vi "Spectrometer_hittite.vi"(6 "ESR_stack_ref":refnum<vi>, 8 "current_run_ref":refnum<vi>, 9 "generator_enable":bool, 10 "sweep_parameters":T2={"Repetitions"=1, "Power dBm"=5.999999061226845, "Freq Start [Hz]"=2800000000.0, "Freq Stop [Hz]"=3000000000.0, "Step size [Hz]"=2500000.0, "Dwell Time [s]"=0.09999999974525053} {"Dwell Time [s]" format="%.3f"; "Step size [Hz]" format="%.2p"; "Freq Stop [Hz]" format="%.2p"; "Freq Start [Hz]" format="%.2p"; "Power dBm" format="%.2f"; "Repetitions" min=1 max=1000 step=1}, 11 "position_xyz":T1 {"Position Z" min=0.0 max=10.0 step=0.001 format="%.3f"; "Position Y" min=-10.0 max=10.0 step=0.1 format="%.3f"; "Position X" min=-10.0 max=10.0 step=0.1 format="%.3f"}) -> ()   [LabVIEW 2014]
uses:
  <vilib>/DAQmx/write.llb/DAQmx Write (Analog 1D DBL NChan 1Samp).vi
  <vilib>/DAQmx/write.llb/DAQmx Write (Digital Bool 1Line 1Point).vi
  <vilib>/Analysis/baseanly.llb/Vector x A.vi
  <vilib>/DAQmx/miscellaneous.llb/DAQmx Fill In Error Info.vi
  GLOBAL_VAR.vi
  <vilib>/Analysis/Matrix/Numeric/Conversions/Array To Matrix - RA2.vi
  <instrlib>/HMC-T2100/Private/Go to Local.vi
  <vilib>/DAQmx/create/channels.llb/DAQmx Create Channel (CO-Pulse Generation-Ticks).vi
  <vilib>/DAQmx/create/channels.llb/DAQmx Create Channel (AO-Voltage-Basic).vi
  <vilib>/DAQmx/configure/trigger.llb/DAQmx Start Trigger (Digital Edge).vi
  <instrlib>/HMC-T2100/Private/Source output off.vi
  <instrlib>/HMC-T2100/Private/Source output ON.vi
  <instrlib>/HMC-T2100/HMC-T2100.lvlib
  <resource>/objmgr/daqmx.rc
  <vilib>/Analysis/NI_AALBase.lvlib
  <vilib>/Analysis/Matrix/NI_Matrix.lvlib
panel:
  out "File name":string
  in  "Save":bool
  in  "Stop":bool
  out "Run":i32=100
  out "Remain":i32
  out "Intensity Graph":ext[][](graph)
  out "Histogram":cluster{ext[], ext[]}[](graph)=[{[2700000000.0, 2702500000.0, 2705000000.0, 2707500000.0, 2710000000.0, 2712500000.0, 2715000000.0, 2717500000.0, 2720000000.0, 2722500000.0, 2725000000.0, 2727500000.0, 2730000000.0, 2732500000.0, 2735000000.0, 2737500000.0, 2740000000.0, 2742500000.0, 2745000000.0, 2747500000.0, 2750000000.0, 2752500000.0, 2755000000.0, 2757500000.0, 2760000000.0, 2762500000.0, 2765000000.0, 2767500000.0, 2770000000.0, 2772500000.0, 2775000000.0, 2777500000.0, 2780000000.0, 2782500000.0, 2785000000.0, 2787500000.0, 2790000000.0, 2792500000.0, 2795000000.0, 2797500000.0, 2800000000.0, 2802500000.0, 2805000000.0, 2807500000.0, 2810000000.0, 2812500000.0, 2815000000.0, 2817500000.0, 2820000000.0, 2822500000.0, 2825000000.0, 2827500000.0, 2830000000.0, 2832500000.0, 2835000000.0, 2837500000.0, 2840000000.0, 2842500000.0, 2845000000.0, 2847500000.0, 2850000000.0, 2852500000.0, 2855000000.0, 2857500000.0, 2860000000.0, 2862500000.0, 2865000000.0, 2867500000.0, 2870000000.0, 2872500000.0, 2875000000.0, 2877500000.0, 2880000000.0, 2882500000.0, 2885000000.0, 2887500000.0, 2890000000.0, 2892500000.0, 2895000000.0, 2897500000.0, 2900000000.0, 2902500000.0, 2905000000.0, 2907500000.0, 2910000000.0, 2912500000.0, 2915000000.0, 2917500000.0, 2920000000.0, 2922500000.0, 2925000000.0, 2927500000.0, 2930000000.0, 2932500000.0, 2935000000.0, 2937500000.0, 2940000000.0, 2942500000.0, 2945000000.0, 2947500000.0, 2950000000.0, 2952500000.0, 2955000000.0, 2957500000.0, 2960000000.0, 2962500000.0, 2965000000.0, 2967500000.0, 2970000000.0, 2972500000.0, 2975000000.0, 2977500000.0, 2980000000.0, 2982500000.0, 2985000000.0, 2987500000.0, 2990000000.0, 2992500000.0, 2995000000.0, 2997500000.0, 3000000000.0], [26841.121559672197128, 27464.174520667373477, 27576.32405364650522, 29408.099758972323686, 27638.629349746022854, 27576.32405364650522, 27638.629349746022854, 27651.09040896592638, 28398.753962160138, 28311.526547620813311, 28236.76019230139215, 27912.772652583900449, 27850.467356484382814, 27875.389474924189868, 28174.454896201874515, 28697.819383437822648, 28685.35832421791912, 28535.825613579076798, 28809.968916416954391, 29046.729041595121403, 28647.975146558208541, 28523.36455435917327, 28062.305363222742772, 28174.454896201874515, 28473.520317479559163, 27738.31782350525107, 28423.676080599945054, 29133.956456134446093, 28859.8131532965685, 27638.629349746022854, 29133.956456134446093, 27763.239941945058124, 27352.024987688241733, 27439.252402227566423, 28822.429975636857918, 27526.479816766891112, 28548.286672798980325, 27838.006297264479286, 28847.352094076664972, 28884.735271736375553, 29271.02810755338489, 28884.735271736375553, 27289.7196915887241, 28971.962686275700243, 28336.448666060620365, 28548.286672798980325, 27975.077948683418082, 27763.239941945058124, 29470.405055071841321, 28822.429975636857918, 28087.227481662549826, 28286.604429181006259, 27352.024987688241733, 27401.869224567855841, 28398.753962160138, 29308.411285213095471, 28485.98137669946269, 28585.669850458690906, 28710.280442657726175, 28236.76019230139215, 28311.526547620813311, 27576.32405364650522, 27302.180750808627625, 28299.065488400909786, 26878.504737331907709, 28809.968916416954391, 29420.560818192227213, 28859.8131532965685, 27750.778882725154597, 28535.825613579076798, 28398.753962160138, 28261.682310741199204, 28947.040567835893189, 28361.370784500427419, 28785.046797977147337, 28610.59196889849796, 27476.635579887277004, 28062.305363222742772, 28311.526547620813311, 28809.968916416954391, 28647.975146558208541, 28112.14960010235688, 28822.429975636857918, 27738.31782350525107, 28199.377014641681569, 28510.903495139269744, 27451.71346144746995, 28074.766422442646299, 27725.856764285347543, 28635.514087338305014, 28834.891034856761445, 27376.947106128048787, 29096.573278474735512, 28274.143369961102731, 29034.267982375217876, 28560.747732018883852, 27277.258632368820573, 28884.735271736375553, 28049.844304002839245, 27975.077948683418082, 26965.732151871232396, 28809.968916416954391, 28000.000067123225136, 27127.725921729978248, 28037.383244782935718, 28000.000067123225136, 27277.258632368820573, 27800.623119604768705, 28087.227481662549826, 27501.557698327084058, 26778.816263572679492, 26429.906605415380737, 27526.479816766891112, 26442.367664635284264, 26479.750842294994845, 27775.701001164961651, 27040.498507190653559, 26429.906605415380737, 27750.778882725154597, 27464.174520667373477, 27925.233711803803976]}, {[2700000000.0, 2702500000.0, 2705000000.0, 2707500000.0, 2710000000.0, 2712500000.0, 2715000000.0, 2717500000.0, 2720000000.0, 2722500000.0, 2725000000.0, 2727500000.0, 2730000000.0, 2732500000.0, 2735000000.0, 2737500000.0, 2740000000.0, 2742500000.0, 2745000000.0, 2747500000.0, 2750000000.0, 2752500000.0, 2755000000.0, 2757500000.0, 2760000000.0, 2762500000.0, 2765000000.0, 2767500000.0, 2770000000.0, 2772500000.0, 2775000000.0, 2777500000.0, 2780000000.0, 2782500000.0, 2785000000.0, 2787500000.0, 2790000000.0, 2792500000.0, 2795000000.0, 2797500000.0, 2800000000.0, 2802500000.0, 2805000000.0, 2807500000.0, 2810000000.0, 2812500000.0, 2815000000.0, 2817500000.0, 2820000000.0, 2822500000.0, 2825000000.0, 2827500000.0, 2830000000.0, 2832500000.0, 2835000000.0, 2837500000.0, 2840000000.0, 2842500000.0, 2845000000.0, 2847500000.0, 2850000000.0, 2852500000.0, 2855000000.0, 2857500000.0, 2860000000.0, 2862500000.0, 2865000000.0, 2867500000.0, 2870000000.0, 2872500000.0, 2875000000.0, 2877500000.0, 2880000000.0, 2882500000.0, 2885000000.0, 2887500000.0, 2890000000.0, 2892500000.0, 2895000000.0, 2897500000.0, 2900000000.0, 2902500000.0, 2905000000.0, 2907500000.0, 2910000000.0, 2912500000.0, 2915000000.0, 2917500000.0, 2920000000.0, 2922500000.0, 2925000000.0, 2927500000.0, 2930000000.0, 2932500000.0, 2935000000.0, 2937500000.0, 2940000000.0, 2942500000.0, 2945000000.0, 2947500000.0, 2950000000.0, 2952500000.0, 2955000000.0, 2957500000.0, 2960000000.0, 2962500000.0, 2965000000.0, 2967500000.0, 2970000000.0, 2972500000.0, 2975000000.0, 2977500000.0, 2980000000.0, 2982500000.0, 2985000000.0, 2987500000.0, 2990000000.0, 2992500000.0, 2995000000.0, 2997500000.0, 3000000000.0], [27662.305362263847, 27614.704116043806, 27558.75396014644, 27479.62623410005, 27635.264863756656, 27635.514084941045, 27523.73838373851, 27614.704116043802, 27583.17763621744, 27571.58885114293, 27593.520315369973, 27605.109100444486, 27505.545237277456, 27540.685424277577, 27573.831841802512, 27521.74461426332, 27747.788228512374, 27553.395704681883, 27408.099754177805, 27507.040564383846, 27553.769536458476, 27450.09352374888, 27547.16517507192, 27590.529661157172, 27485.98137430221, 27331.838071751987, 27460.06237112481, 27420.436202805507, 27402.99071989765, 27434.64181031619, 27576.697885423117, 27476.38635870286, 27470.654271461714, 27460.311592309215, 27451.962682631867, 27448.722807234688, 27469.781997316335, 27462.056140599987, 27364.23682572375, 27414.081062603364, 27456.573274543232, 27499.688539444087, 27488.598196738385, 27439.252402227583, 27451.215019078678, 27574.45489476352, 27513.894146954794, 27562.741499096825, 27559.377013107456, 27384.42374165998, 27576.074832462113, 27480.747729429848, 27504.423741947663, 27448.099754273695, 27508.90972326683, 27439.50162341197, 27397.383243248685, 27424.54835234809, 27331.21501879102, 27477.258632848276, 27459.68853934821, 27434.267978539607, 27381.05925567063, 27417.07171681613, 27347.912838145676, 27456.82249572762, 27392.398819560723, 27427.539006560855, 27402.86610930546, 27384.79757343659, 27482.86610949723, 27504.049910171063, 27508.037449121424, 27430.778881958024, 27495.202558124915, 27442.367667032533, 27426.16829004667, 27367.60131171313, 27402.616888121054, 27600.00006616432, 27539.68853953999, 27533.58262052224, 27462.305361784383, 27564.361436795392, 27572.087293511737, 27503.55146780227, 27476.137137518494, 27474.766421004293, 27580.560813781274, 27579.813150228085, 27592.024988263576, 27505.296016093063, 27570.84118758975, 27614.953337228195, 27611.215019462234, 27484.236826011424, 27503.925299578863, 27544.54835263575, 27602.616888600503, 27550.903492837893, 27593.769536554377, 27516.63557998317, 27611.962683015438, 27551.028103430108, 27655.701000877292, 27659.688539827646, 27578.5670443061, 27729.59508205134, 27610.093524132444, 27489.968913252564, 27615.202558412602, 27486.479816671, 27421.059255766515, 27418.56704392252, 27449.221249603488, 27600.996950901917, 27543.92529967475, 27425.17140530909, 27466.04367955036, 27523.987604922913, 27501.183866550484]}]
  in  "start":bool
  in  "stop":bool
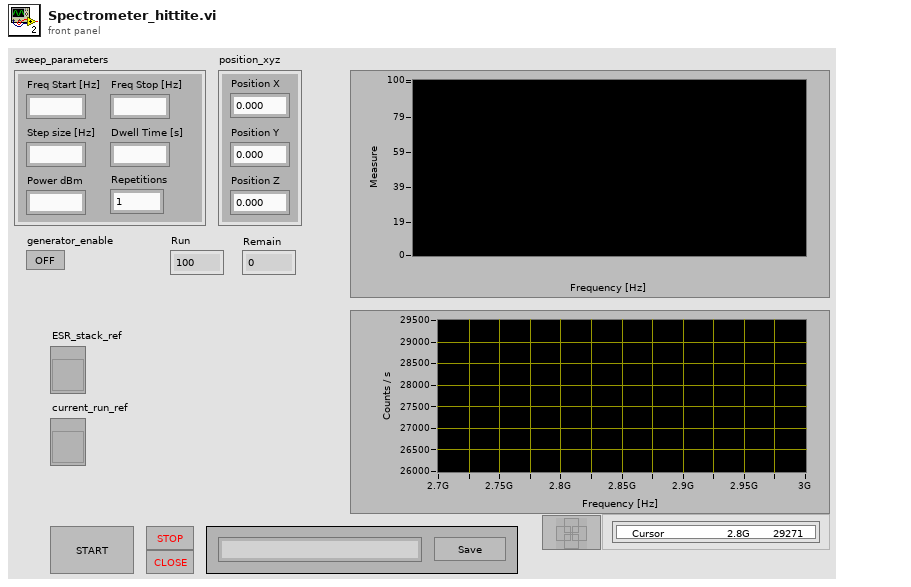
[diagram p1: front panel]
types:
  T1 = cluster{"Position X":dbl, "Position Y":dbl, "Position Z":dbl}
  T2 = cluster{"Repetitions":i32, "Power dBm":ext, "Freq Start [Hz]":ext, "Freq Stop [Hz]":ext, "Step size [Hz]":ext, "Dwell Time [s]":ext}
  T3 = enum16{"stand-by", "init", "config", "acquisition", "processing", "close", "Set Variables", "Error Check"}
  T4 = enum16{"stand-by", "init", "config", "acquisition", "processing", "close", "Set Variables"}
  T5 = cluster{"Baud Rate":u32, "Parity":u16, "Data Bits":u16, "Stop Bits":u16, "Flow Control":u16}
  T6 = typedef "NI_Matrix.lvlib/RealMatrix.ctl" = dbl[][]
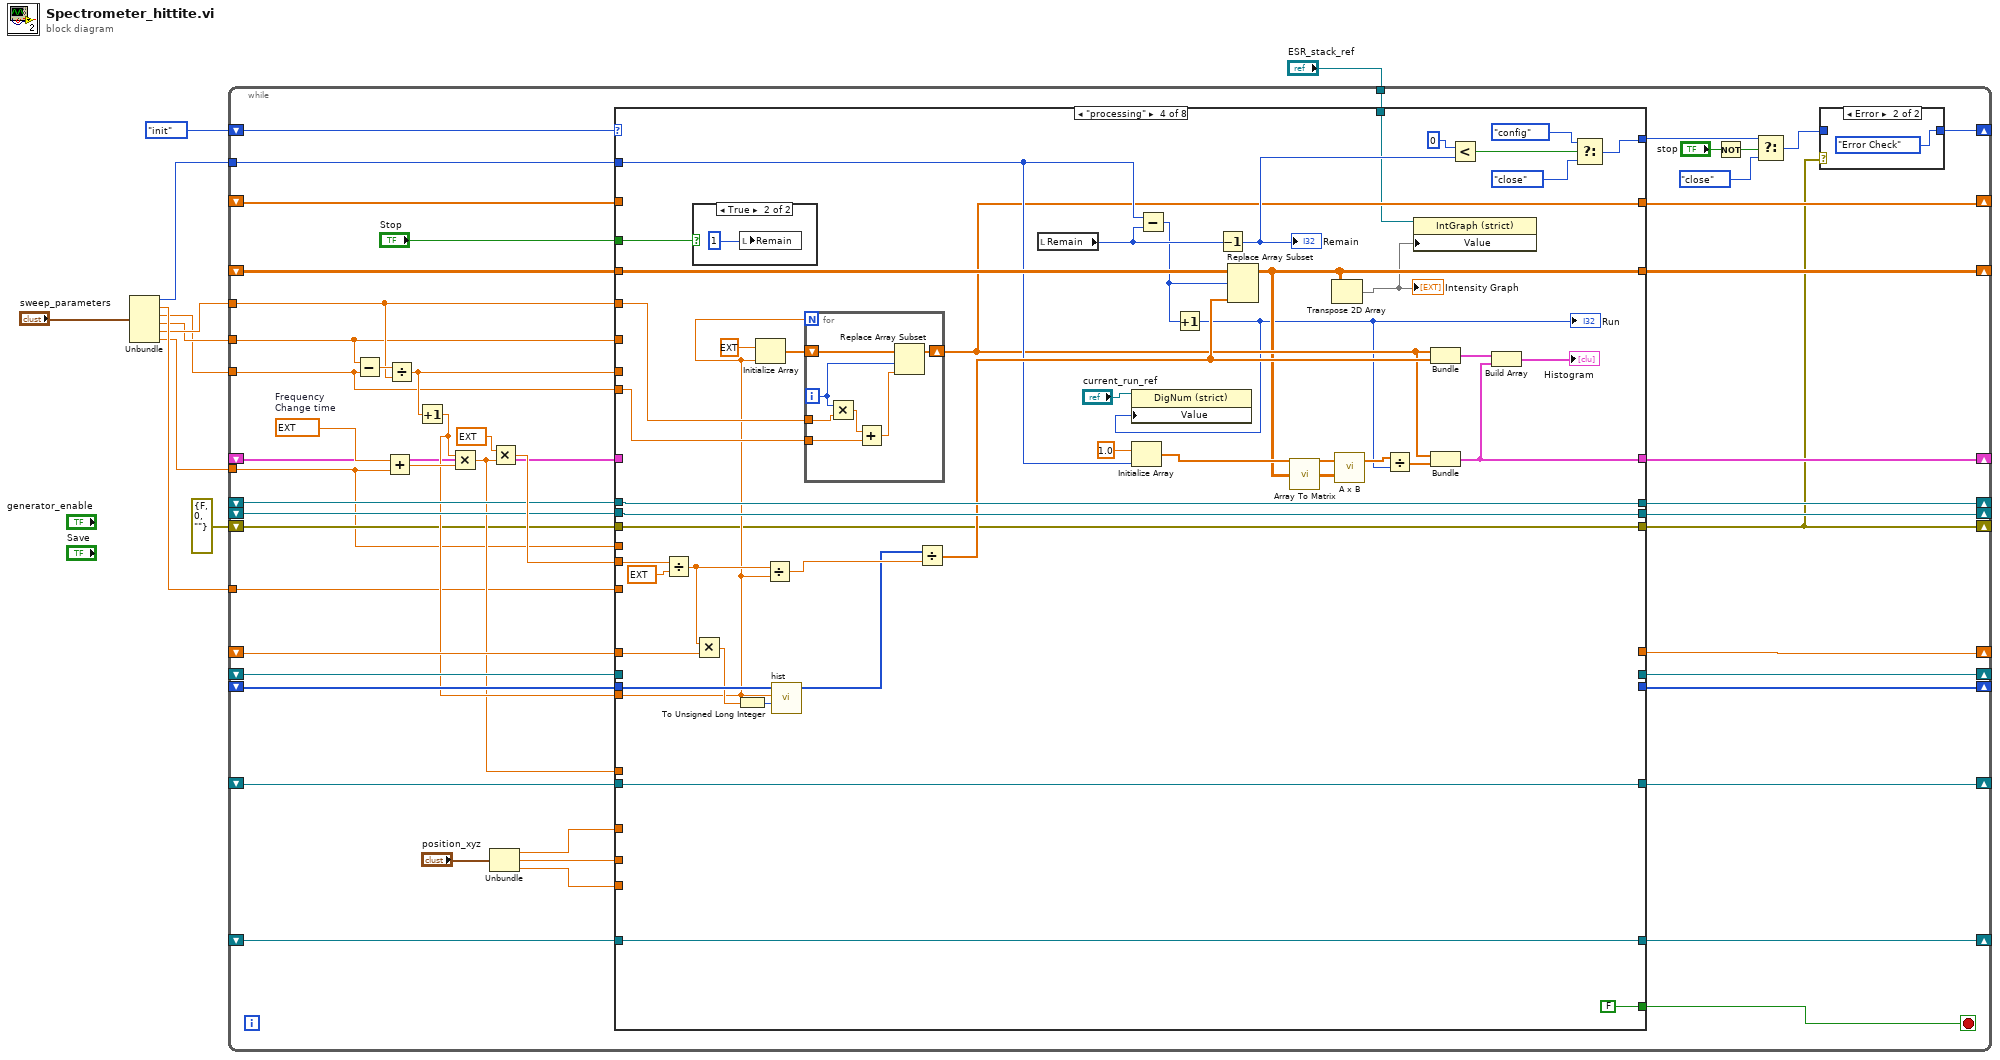
[diagram p0: block diagram]
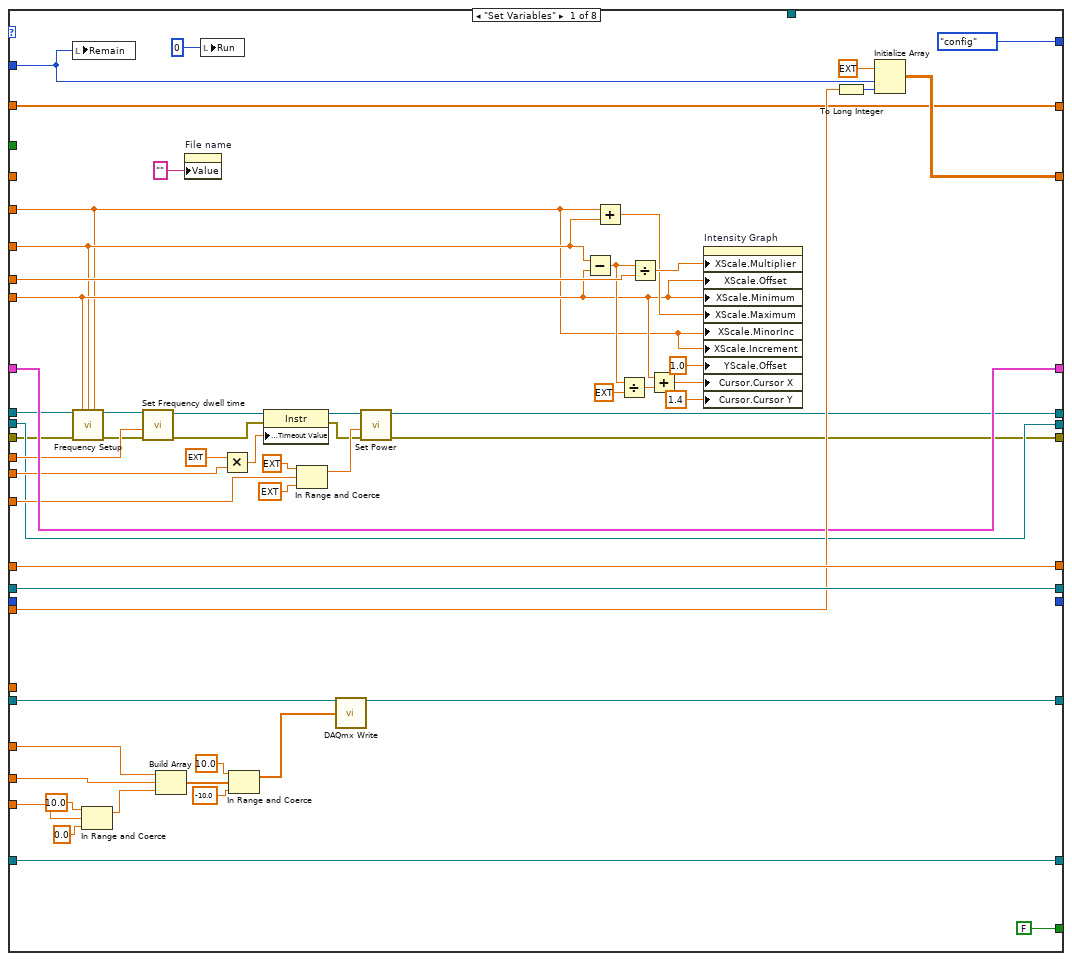
[diagram p3: hidden frame]
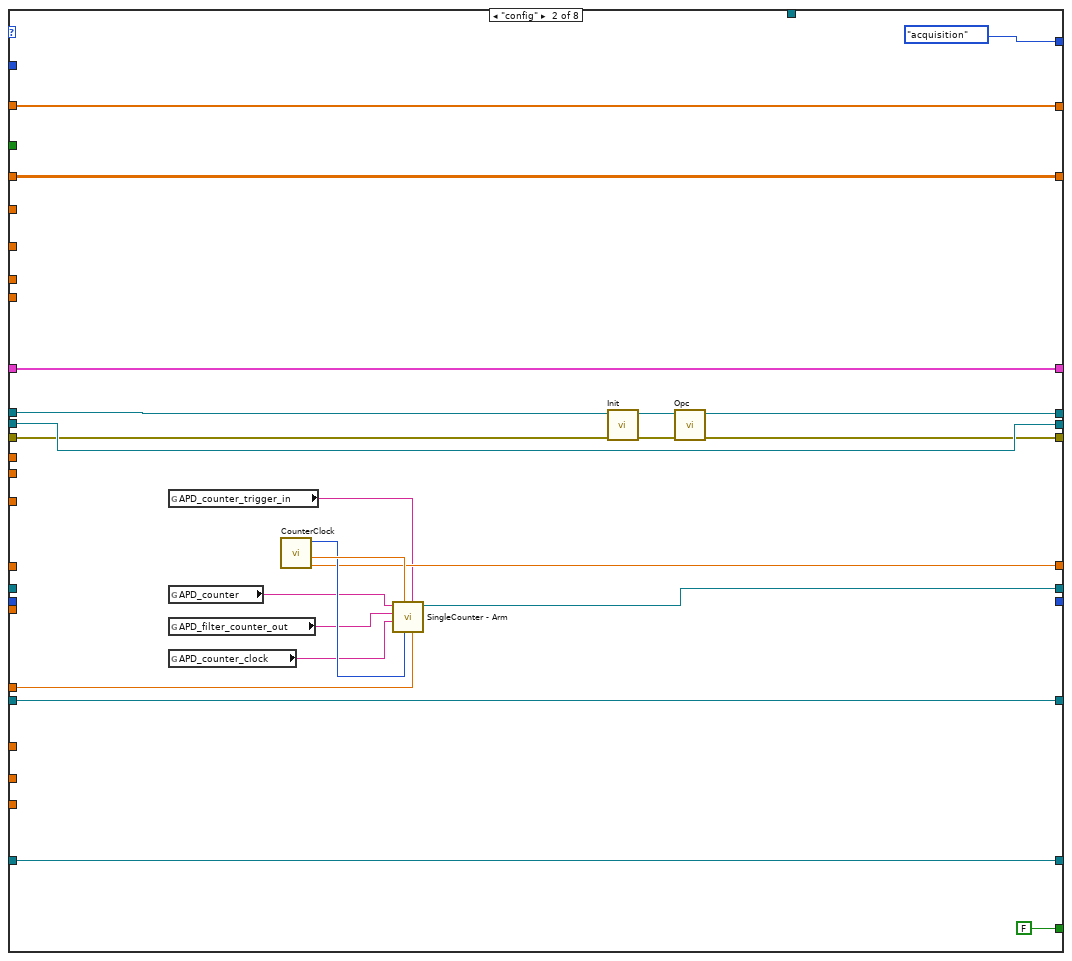
[diagram p4: hidden frame]
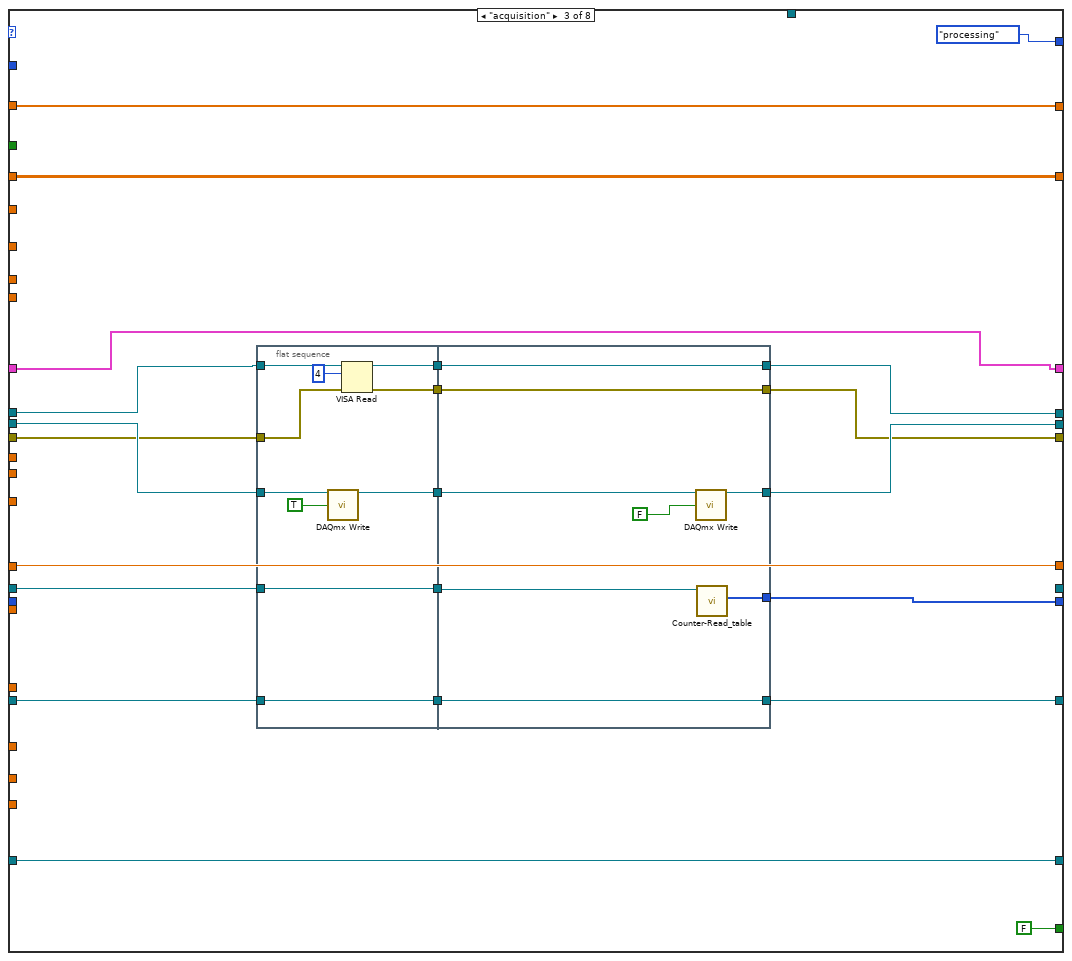
[diagram p5: hidden frame]
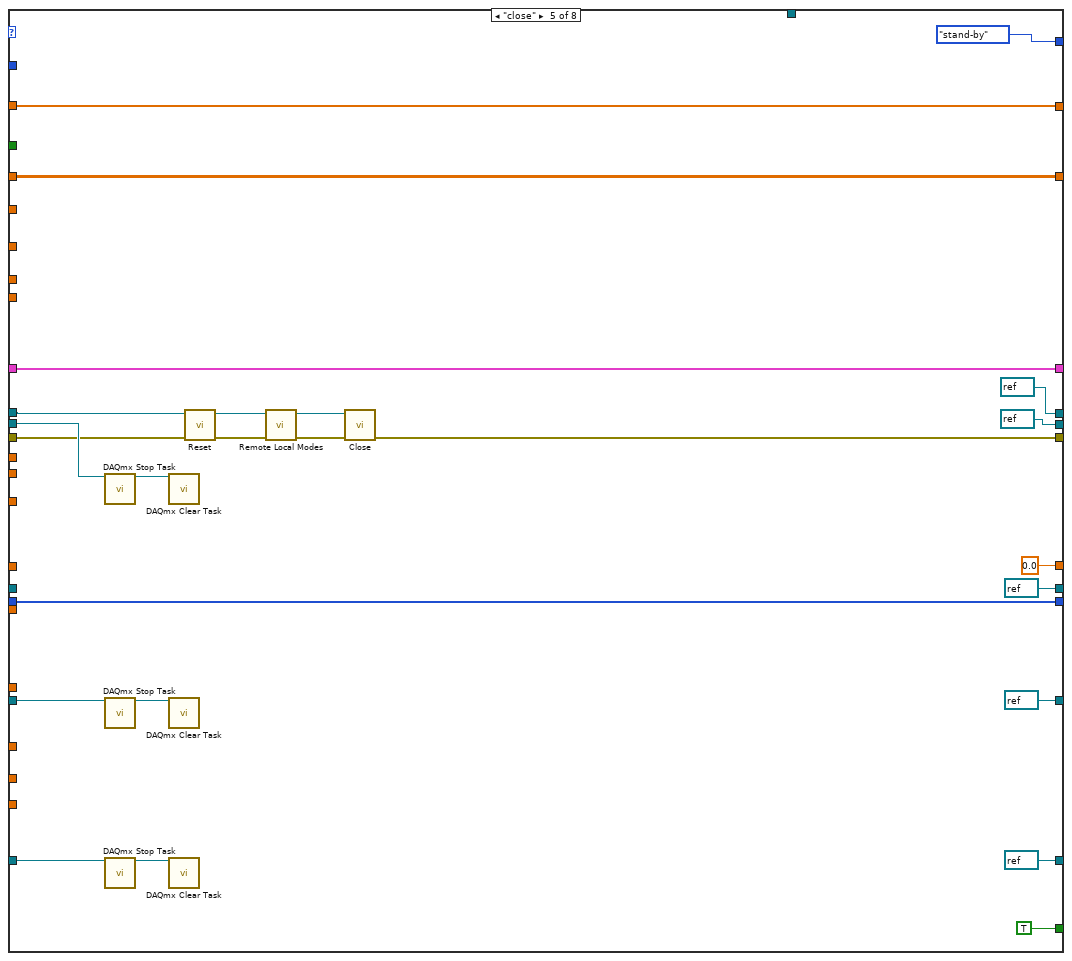
[diagram p7: hidden frame]
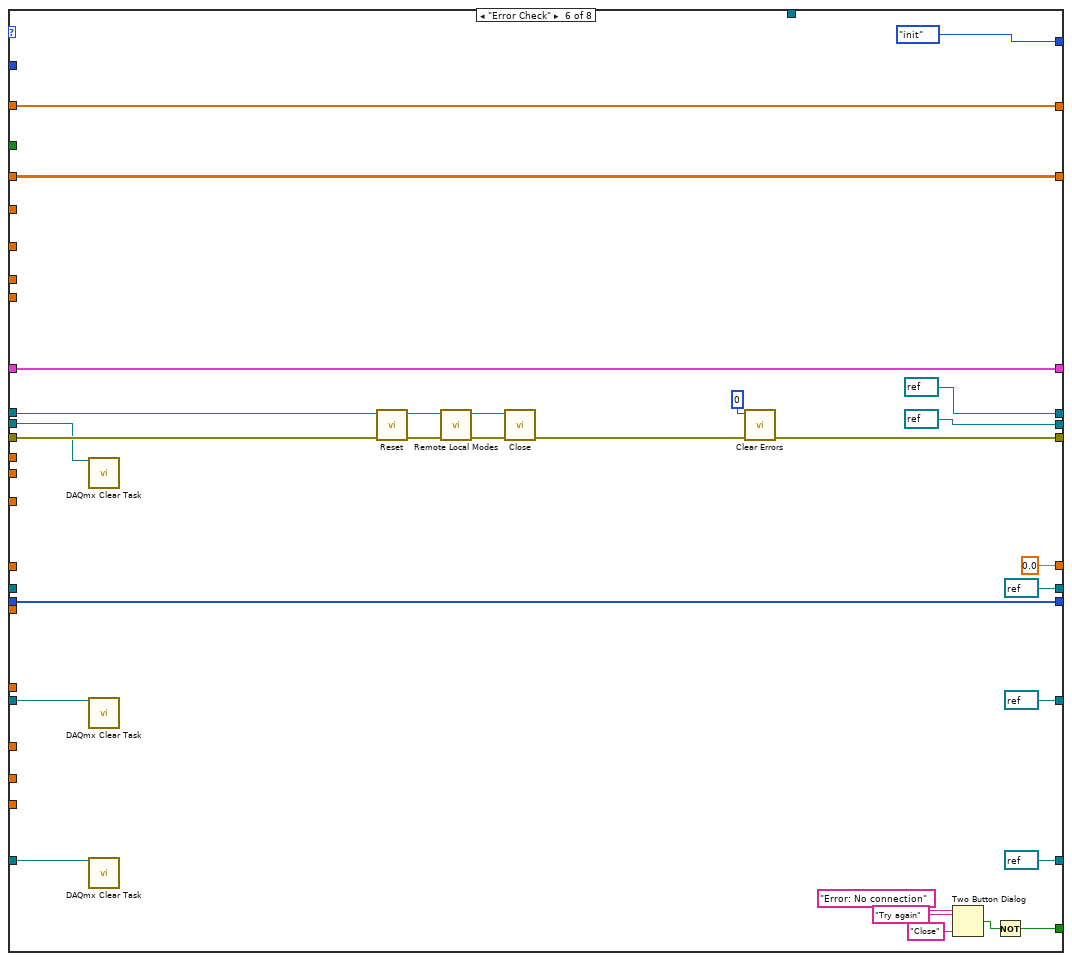
[diagram p8: hidden frame]
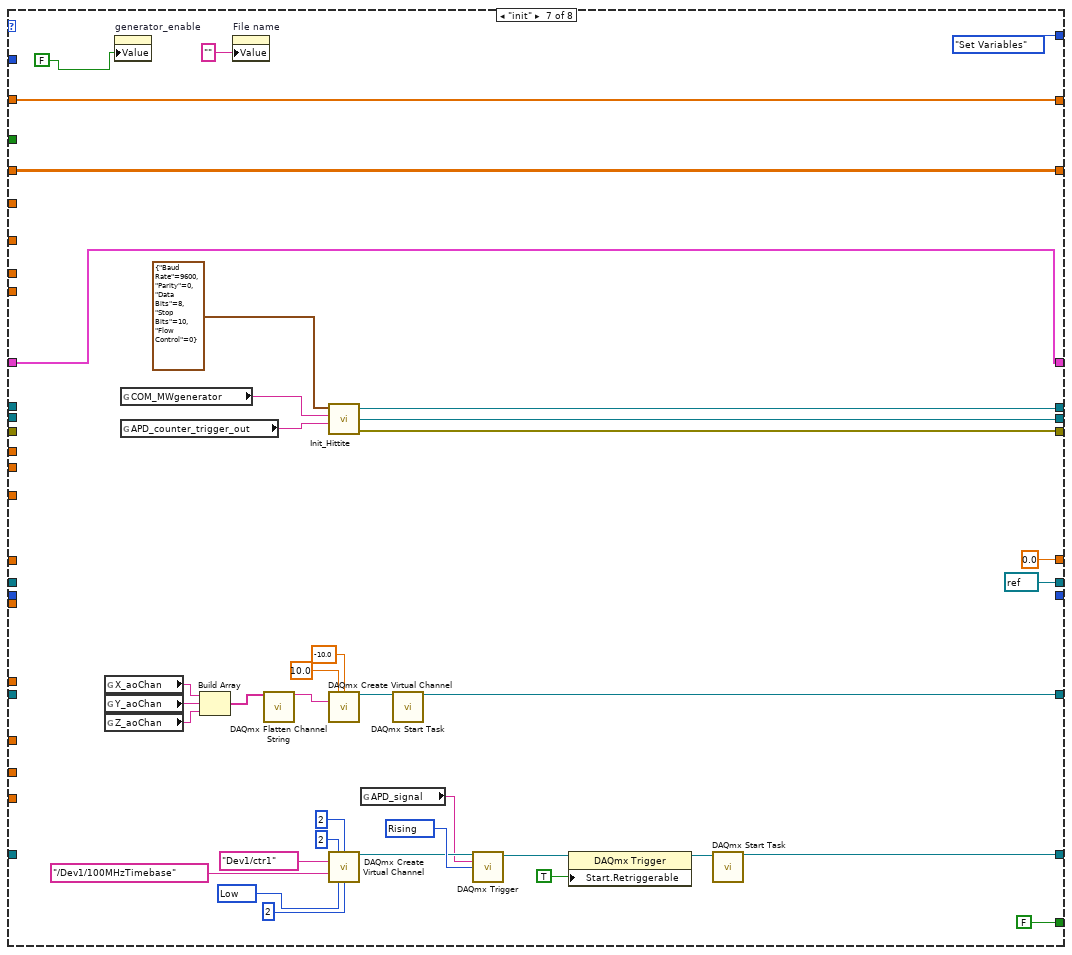
[diagram p9: hidden frame]
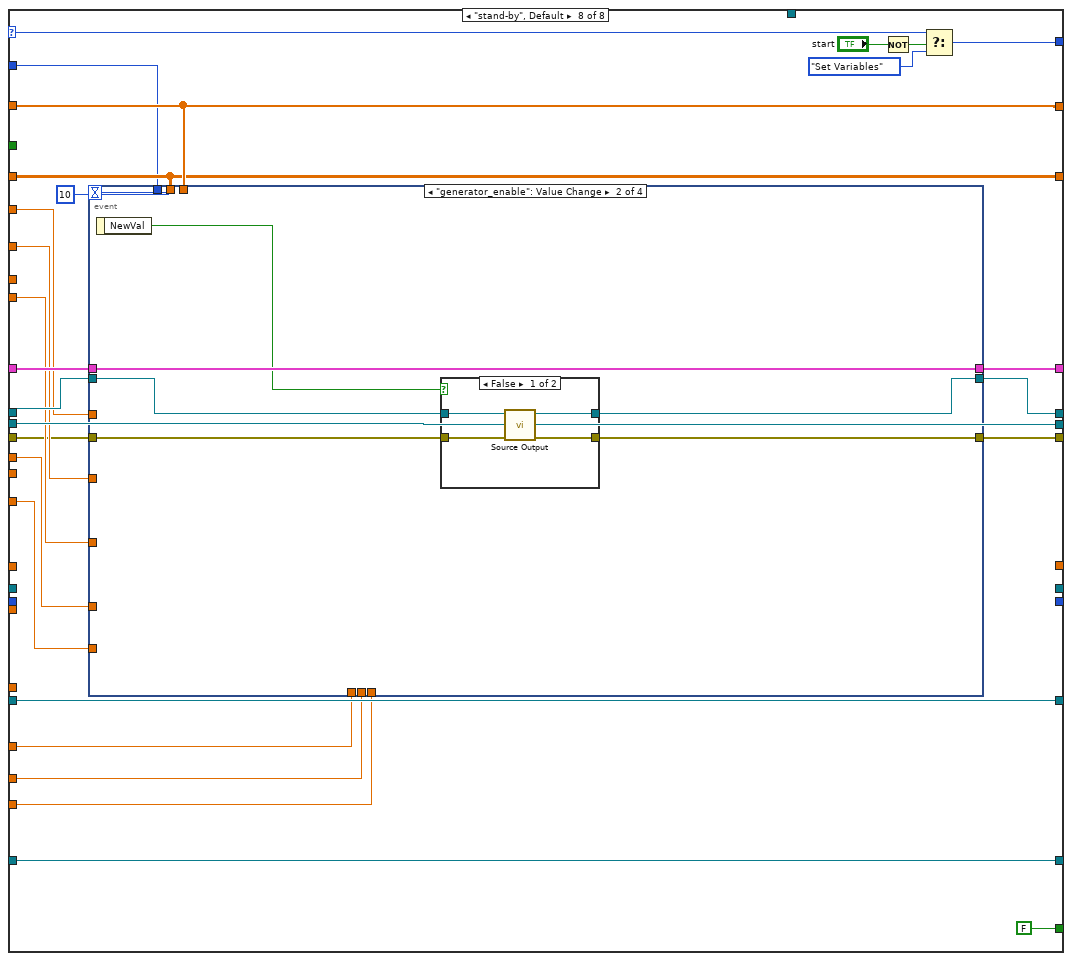
[diagram p10: hidden frame]
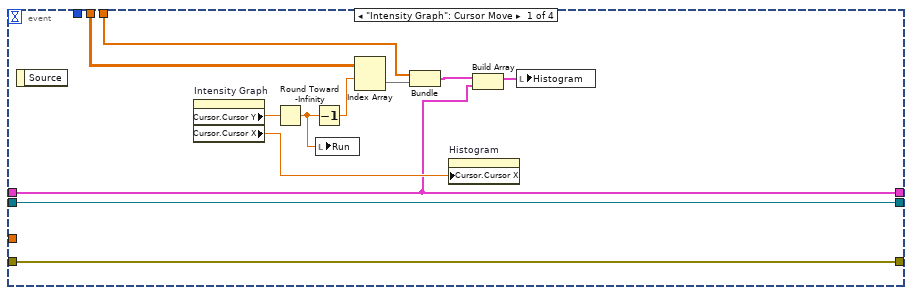
[diagram p11: hidden frame]
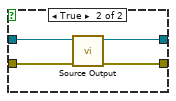
[diagram p12: hidden frame]
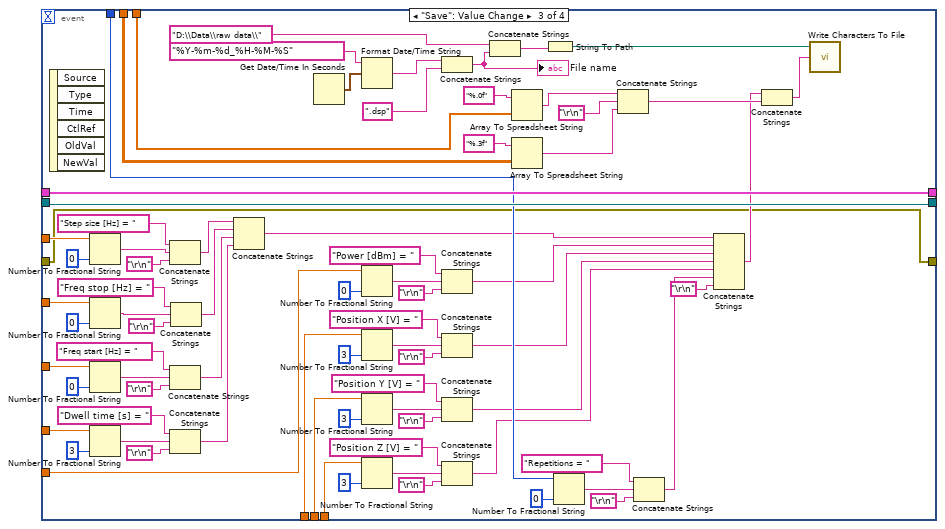
[diagram p13: hidden frame]
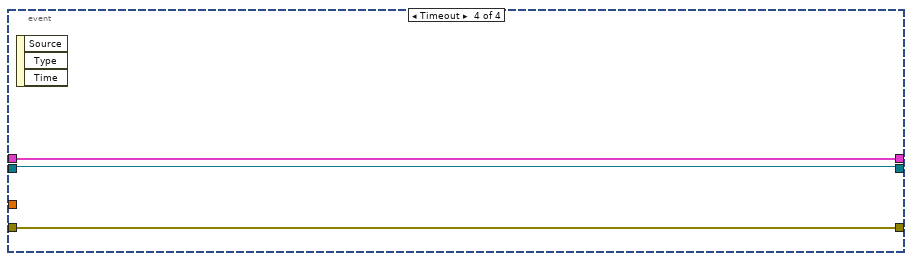
[diagram p14: hidden frame]
diagram:
  n1 = Unbundle("sweep_parameters") -> ("Repetitions"=w7:i32, "Power dBm"=w6:ext, "Freq Start [Hz]"=w2:ext, "Freq Stop [Hz]"=w3:ext, "Step size [Hz]"=w4:ext, "Dwell Time [s]"=w5:ext)
  n2 = while {
    shift-right: [w24] -> _
    shift-left: T3."init" -> [w60]
    shift-right: [w55] -> _
    shift-left: _ -> [w53]
    shift-right: [w54] -> _
    shift-left: _ -> [w52]
    shift-right: [w51] -> _
    shift-left: _ -> [w50]
    shift-right: [w49] -> _
    shift-left: _ -> [w48]
    shift-right: [w43] -> _
    shift-left: _ -> [w42]
    shift-right: [w27] -> _
    shift-left: _ -> [w38]
    shift-right: [w35] -> _
    shift-left: _ -> [w37]
    shift-right: [w34] -> _
    shift-left: _ -> [w33]
    shift-right: [w31] -> _
    shift-left: _ -> [w30]
    shift-right: [w29] -> _
    shift-left: _ -> [w28]
    shift-right: [w22] -> _
    shift-left: errorcluster {"status"=FALSE, "code"=0, "source"=""} ("error out") -> [w25]
    tunnel: w7 -> [w17]
    tunnel: w6 -> [w16]
    tunnel: w5 -> [w15]
    tunnel: w4 -> [w14]
    tunnel: w3 -> [w13]
    tunnel: w2 -> [w12]
    tunnel: "ESR_stack_ref" -> [w11]
    stop <- w44 stop-if-true
    w58 = ext 0.0002500000118743628  # Frequency Change time
    n3 = Subtract(x=w13, y=w12) -> (x-y=w59:ext)
    n4 = Add(x=w58, y=w15) -> (x+y=w57:ext)
    n5 = Divide(x=w59, y=w14) -> (x/y=w39:ext)
    n6 = Increment(x=w39) -> (x+1=w40:ext)
    n7 = Multiply(x=w40, y=w57) -> (x*y=w32:ext)
    n8 = Unbundle("position_xyz") -> ("Position X"=w20:dbl, "Position Y"=w18:dbl, "Position Z"=w19:dbl)
    n9 = Multiply(x=ext 1000.0 ("y"), y=w32) -> (x*y=w56:ext)
    n10 = case shown="\"processing\"" w60 {
      selector: w60 -> [_ _ _ _ _ _ _ w353]
      tunnel: [T4."config" T4."acquisition" T4."processing" w212 T4."stand-by" T3."init" T3."Set Variables" w352] -> w45
      tunnel: [w69 w140 w159 w222 refnum<visa-resource-name> refnum ("T2100 Address OUT") refnum<visa-resource-name> refnum ("T2100 Address Out") w299 w338] -> w55
      tunnel: [w71 w141 w160 w221 refnum<k21> refnum ("Trigger_out") refnum<k21> refnum ("task out") w298 w350] -> w54
      tunnel: w53 -> [w85 w127 w162 w222 w255 w273 _ w339]
      tunnel: w52 -> [w71 w141 w161 w221 w261 w265 _ w350]
      tunnel: w14 -> [w78 _ _ w220 _ _ _ w327]
      tunnel: w13 -> [w79 _ _ _ _ _ _ w337]
      tunnel: w12 -> [w80 _ _ w205 _ _ _ w336]
      tunnel: w56 -> [w76 _ _ w216 _ _ _ _]
      tunnel: w15 -> [w77 _ _ _ _ _ _ w335]
      tunnel: [w115 w136 _ _ refnum<k21> refnum ("task out") refnum<k21> refnum ("task out") refnum<k21> refnum ("task out") _] -> w51
      tunnel: w50 -> [w115 _ w157 _ _ _ _ _]
      tunnel: [_ _ w156 _ w237 w262 _ _] -> w49
      tunnel: w48 -> [_ _ _ w227 w237 w262 _ _]
      tunnel: [FALSE FALSE FALSE FALSE TRUE w282 FALSE FALSE] -> w44
      tunnel: [w114 w135 w154 _ 0.0 ("Counter clock rate divided by prescaler") 0.0 ("Counter clock rate divided by prescaler") 0.0 ("Counter clock rate divided by prescaler") _] -> w43
      tunnel: w42 -> [w114 _ w154 w225 _ _ _ _]
      tunnel: w40 -> [w111 _ _ w200 _ _ _ _]
      tunnel: w39 -> [w110 _ _ _ _ _ _ _]
      tunnel: w16 -> [w72 _ _ _ _ _ _ w334]
      tunnel: w20 -> [w90 _ _ _ _ _ _ w333]
      tunnel: w38 -> [w97 w128 w152 w217 w257 w264 _ w348]
      tunnel: w18 -> [w89 _ _ _ _ _ _ w332]
      tunnel: w19 -> [w88 _ _ _ _ _ _ w331]
      tunnel: w17 -> [w101 _ _ w197 _ _ _ w330]
      tunnel: w37 -> [_ w134 w150 w209 w254 w267 w325 w343]
      tunnel: [w113 w134 w150 w189 w254 w267 w325 w343] -> w35
      tunnel: [w102 w132 w148 w195 w252 w268 w324 w345] -> w34
      tunnel: w33 -> [w102 w132 w148 _ w252 w268 w324 w345]
      tunnel: w32 -> [_ w131 _ _ _ _ _ _]
      tunnel: [w99 w130 w147 w202 refnum<k21> refnum ("task out") refnum<k21> refnum ("task out") w307 w342] -> w31
      tunnel: w30 -> [w99 w130 w147 w202 w250 w263 _ w342]
      tunnel: [w98 w129 w146 w191 w249 w266 w323 w340] -> w29
      tunnel: w28 -> [w98 w129 w146 _ w249 w266 w323 w341]
      tunnel: [w96 w128 w151 w217 refnum<k21> refnum ("task out") refnum<k21> refnum ("task out") w301 w348] -> w27
      tunnel: "Stop" -> [_ _ _ w190 _ _ _ _]
      tunnel: [w64 w124 w144 w188 w244 w287 w300 w328] -> w22
      tunnel: w25 -> [w63 w126 w145 w188 w247 w275 _ w329]
      tunnel: w11 -> [_ _ _ w184 _ _ _ _]
      frame "Set Variables" {
        n11 = local write "Remain"(w101) -> ()
        n12 = call <instrlib>:"Frequency Setup.vi"("T2100 Address In"=w85, "Frequency Start"=w80, "Frequency Stop"=w79, "Frequency Step"=w78, "error in"=w63) -> ("T2100 Address Out"=w84:refnum<visa-resource-name>, "error out"=w67:errorcluster)  [unwired: 9 in]
        n13 = In Range and Coerce(upper limit=10.0, x=w88, lower limit=0.0) -> (coerced(x)=w92:dbl)  [unwired: 1 out]
        n14 = call <instrlib>:"Set Frequency dwell time.vi"("error in"=w67, "Time"=w77, "T2100 Address In"=w84) -> ("error out"=w66:errorcluster, "T2100 Address Out"=w83:refnum<visa-resource-name>)  [unwired: 7 in]
        n15 = Build Array(w90, w89, w92) -> (w91:dbl[])
        n16 = property on="File name" class="Str"("Value"="" ("File name")) -> ()  [unwired: 2 in, 2 out]
        n17 = local write "Run"(0 ("Run")) -> ()
        n18 = Multiply(x=ext 1.100000023841858, y=w76) -> (x*y=w86:ext)
        n19 = In Range and Coerce(upper limit=10.0, x=w91, lower limit=-10.0) -> (coerced(x)=w87:dbl[])  [unwired: 1 out]
        n20 = property class="Instr"(reference=w83, error in=w66, "General Settings:Timeout Value"=w86) -> (reference out=w82:refnum<visa-resource-name>, error out=w65:errorcluster)
        n21 = In Range and Coerce(upper limit=ext 27.0, x=w72, lower limit=ext -36.0) -> (coerced(x)=w73:ext)  [unwired: 1 out]
        n22 = call-poly <vilib>:"DAQmx Write.vi"("task/channels in"=w97, "data"=w87) -> ("task out"=w96:refnum<k21>)  [unwired: 11 in, 2 out]
        n23 = call <instrlib>:"Set Power.vi"("error in"=w65, "RF Power"=w73, "T2100 Address IN"=w82) -> ("error out"=w64:errorcluster, "T2100 Address OUT"=w69:refnum<visa-resource-name>)  [unwired: 7 in]
        n24 = Subtract(x=w79, y=w80) -> (x-y=w107:ext)
        n25 = Add(x=w78, y=w79) -> (x+y=w109:ext)
        n26 = Divide(x=w107, y=ext 2.0) -> (x/y=w103:ext)
        n27 = Divide(x=w107, y=w110) -> (x/y=w112:ext)
        n28 = Add(x=w80, y=w103) -> (x+y=w104:ext)
        n29 = property on="Intensity Graph" class="IntGraph (strict)"("XScale.Multiplier"=w112, "XScale.Offset"=w80, "XScale.Minimum"=w80, "XScale.Maximum"=w109, "XScale.MinorInc"=w78, "XScale.Increment"=w78, "YScale.Offset"=1.0 ("Y Scale.Offset and Multiplier:Offset"), "Cursor.Cursor X"=w104, "Cursor.Cursor Y"=1.4 ("Cursor.Cursor Position:Cursor Y")) -> ()  [unwired: 2 in, 2 out]
        n30 = To Long Integer(number=w111) -> (32bit integer=w117:i32)
        n31 = Initialize Array(ext 0.0 ("element"), w101, w117) -> (w113:ext[][])
      }
      frame "config" {
        n32 = global read "GLOBAL_VAR.vi" "APD_counter_trigger_in"() -> (w123:tag)
        n33 = global read "GLOBAL_VAR.vi" "APD_counter"() -> (w122:tag)
        n34 = global read "GLOBAL_VAR.vi" "APD_filter_counter_out"() -> (w120:tag)
        n35 = global read "GLOBAL_VAR.vi" "APD_counter_clock"() -> (w121:tag)
        n36 = call "CounterClock.vi"() -> ("Counter clock rate divided by prescaler"=w135:dbl, "Counter clock rate"=w138:dbl, "CI.Prescaler"=w137:u32)  [unwired: 8 in, 1 out]
        n37 = call "SingleCounter - Arm.vi"("Duration"=w131, "Trigger Source"=w123, "CI.Prescaler"=w137, "Sampling Rate"=w138, "Clock Source"=w121, "External Timing Source"=w120, "counter"=w122) -> ("task out"=w136:refnum<k21>)  [unwired: 3 in, 1 out]
        n38 = call "Init.vi"("error in"=w126, "VISA resource name"=w127) -> ("error out"=w125:errorcluster, "VISA resource name out"=w142:refnum<visa-resource-name>)  [unwired: 8 in]
        n39 = call "Opc.vi"("error in"=w125, "VISA resource name"=w142) -> ("error out"=w124:errorcluster, "VISA resource name out"=w140:refnum<visa-resource-name>)  [unwired: 8 in]
      }
      frame "acquisition" {
        n40 = flat-sequence {
          tunnel: w162 -> [w171]
          tunnel: w161 -> [w173]
          tunnel: [w170] -> w164
          tunnel: [w172] -> w163
          tunnel: [w168] -> w158
          tunnel: w157 -> [w168]
          tunnel: [w167] -> w153
          tunnel: w152 -> [w167]
          tunnel: w145 -> [w166]
          tunnel: [w165] -> w143
          tunnel: [w179] -> w160
          tunnel: [w182] -> w159
          tunnel: w164 -> [w182]
          tunnel: w163 -> [w180]
          tunnel: w158 -> [w177]
          tunnel: [w178] -> w156
          tunnel: [w176] -> w151
          tunnel: w153 -> [w176]
          tunnel: [w175] -> w144
          tunnel: w143 -> [w175]
          frame #0 {
            n41 = call-poly <vilib>:"DAQmx Write.vi"("task/channels in"=w173, "data"=TRUE) -> ("task out"=w172:refnum<k21>)  [unwired: 11 in, 2 out]
            n42 = VISA Read(VISA resource name=w171, byte count=u32 4, error in (no error)=w166) -> (VISA resource name out=w170:refnum<visa-resource-name>, error out=w165:errorcluster)  [unwired: 2 out]
          }
          frame #1 {
            n43 = call-poly <vilib>:"DAQmx Write.vi"("task/channels in"=w180, "data"=FALSE) -> ("task out"=w179:refnum<k21>)  [unwired: 11 in, 2 out]
            n44 = call "Counter-Read_table.vi"("task in"=w177) -> ("time tags"=w178:u32[])  [unwired: 9 in, 1 out]
          }
        }
      }
      frame "processing" {
        n45 = Divide(x=w216, y=ext 1000.0) -> (x/y=w215:ext)
        n46 = case shown="True" w190 {
          frame False {
          }
          frame True {
            n47 = local write "Remain"(1) -> ()
          }
        }
        n48 = Multiply(x=w215, y=w225) -> (x*y=w223:ext)
        n49 = To Unsigned Long Integer(number=w223) -> (unsigned 32bit integer=w224:u32)
        n50 = Initialize Array(ext 0.0 ("element"), w200) -> (w218:ext[])
        n51 = Divide(x=w215, y=w200) -> (x/y=w214:ext)
        n52 = call "hist.vi"("#clock cycles"=w224, "#bins"=w200, "counter timetag list"=w227) -> ("histogram"=w213:i32[])  [unwired: 7 in]
        n53 = for {
          N: w200 -> [_]
          tunnel: w220 -> [w232]
          shift-right: [w236] -> w195
          shift-left: w218 -> [w235]
          tunnel: w205 -> [w234]
          i -> [w233]
          n54 = Multiply(x=w233, y=w232) -> (x*y=w231:ext)
          n55 = Add(x=w231, y=w234) -> (x+y=w230:ext)
          n56 = Replace Array Subset(array=w235, new element=w230, index=w233) -> (w236:ext[])
        }
        n57 = Divide(x=w213, y=w214) -> (x/y=w201:ext[])
        n58 = local read "Remain"() -> (w204:i32)
        n59 = Initialize Array(1.0 ("element"), w197) -> (w196:dbl[])
        n60 = Subtract(x=w197, y=w204) -> (x-y=w203:i32)
        n61 = Increment(x=w203) -> (x+1=w185:i32)
        "Run" <- w185
        n62 = property class="DigNum (strict)"(reference="current_run_ref", "Value"=w185) -> ()  [unwired: 1 in, 2 out]
        n63 = Decrement(x=w204) -> (x-1=w206:i32)
        "Remain" <- w206
        n64 = Replace Array Subset(array=w209, new element=w201, index (row)=w203) -> (w189:ext[][])  [unwired: 1 in]
        n65 = call-poly <vilib>:"Array To Matrix.vi"("Real 2D Array"=w189) -> ("Real Matrix"=w199:T6)
        n66 = Transpose 2D Array(2D array=w189) -> (transposed array=w183:ext[][])
        "Intensity Graph" <- w183
        n67 = call-poly <vilib>:"A x B.vi"("Matrix A"=w199, "Vector V'"=w196) -> ("V' x A"=w193:dbl[])  [unwired: 1 out]
        n68 = Divide(x=w193, y=w185) -> (x/y=w194:dbl[])
        n69 = property class="IntGraph (strict)"(reference=w184, "Value"=w183) -> ()  [unwired: 1 in, 2 out]
        n70 = Bundle(w195, w201) -> (w192:cluster{ext[], ext[]})  [unwired: 1 in]
        n71 = Bundle(w195, w194) -> (w191:cluster{ext[], dbl[]})  [unwired: 1 in]
        n72 = Less?(x=0, y=w206) -> (x < y?=w210:bool)
        n73 = Build Array(w192, w191) -> (→"Histogram":cluster{ext[], ext[]}[])
        n74 = Select(t=T4."config", s=w210, f=T4."close") -> (s? t:f=w212:T4)
      }
      frame "close" {
        n75 = call <vilib>:"DAQmx Stop Task.vi"("task/channels in"=w261) -> ("task out"=w260:refnum<k21>)  [unwired: 13 in, 1 out]
        n76 = call <vilib>:"DAQmx Stop Task.vi"("task/channels in"=w257) -> ("task out"=w248:refnum<k21>)  [unwired: 13 in, 1 out]
        n77 = call <vilib>:"DAQmx Stop Task.vi"("task/channels in"=w250) -> ("task out"=w251:refnum<k21>)  [unwired: 13 in, 1 out]
        n78 = call <vilib>:"DAQmx Clear Task.vi"("task in"=w260) -> ()  [unwired: 14 in, 1 out]
        n79 = call <vilib>:"DAQmx Clear Task.vi"("task in"=w248) -> ()  [unwired: 14 in, 1 out]
        n80 = call <vilib>:"DAQmx Clear Task.vi"("task in"=w251) -> ()  [unwired: 14 in, 1 out]
        n81 = call <instrlib>:"Reset.vi"("error in"=w247, "T2100 Address In"=w255) -> ("error out"=w246:errorcluster, "T2100 Address Out"=w256:refnum<visa-resource-name>)  [unwired: 8 out]
        n82 = call-poly <instrlib>:"Remote Local Modes.vi"("error in"=w246, "T2100 Address In"=w256) -> ("error out"=w245:errorcluster, "T2100 Address Out"=w258:refnum<visa-resource-name>)  [unwired: 8 in]
        n83 = call <instrlib>:"Close.vi"("error in (no error)"=w245, "VISA resource name"=w258) -> ("error out"=w244:errorcluster)  [unwired: 9 in]
      }
      frame "Error Check" {
        n84 = call <vilib>:"DAQmx Clear Task.vi"("task in"=w265) -> ()  [unwired: 14 in, 1 out]
        n85 = call <vilib>:"DAQmx Clear Task.vi"("task in"=w264) -> ()  [unwired: 14 in, 1 out]
        n86 = call <vilib>:"DAQmx Clear Task.vi"("task in"=w263) -> ()  [unwired: 14 in, 1 out]
        n87 = call <instrlib>:"Reset.vi"("error in"=w275, "T2100 Address In"=w273) -> ("error out"=w280:errorcluster, "T2100 Address Out"=w279:refnum<visa-resource-name>)  [unwired: 8 out]
        n88 = call-poly <instrlib>:"Remote Local Modes.vi"("error in"=w280, "T2100 Address In"=w279) -> ("error out"=w281:errorcluster, "T2100 Address Out"=w278:refnum<visa-resource-name>)  [unwired: 8 in]
        n89 = call <instrlib>:"Close.vi"("error in (no error)"=w281, "VISA resource name"=w278) -> ("error out"=w274:errorcluster)  [unwired: 9 in]
        n90 = call <vilib>:"Clear Errors.vi"("error in (no error)"=w274, "specific error code to clear (0: all)"=0) -> ("error out"=w287:errorcluster)  [unwired: 4 in, 1 out]
        n91 = Two Button Dialog(message="Error: No connection", 1:"Close" ("F button name (\"Cancel\")"), 2:"Try again" ("T button name (\"OK\")")) -> (T button?=w283:bool)
        n92 = Not(x=w283) -> (.not. x?=w282:bool)
      }
      frame "init" {
        w313 = 10280 items=["Rising"=10280, "Falling"=10171] ("edge")
        w317 = 10214 items=["High"=10192, "Low"=10214] ("idle state")
        n93 = global read "GLOBAL_VAR.vi" "X_aoChan"() -> (w295:tag)
        n94 = global read "GLOBAL_VAR.vi" "Y_aoChan"() -> (w294:tag)
        n95 = global read "GLOBAL_VAR.vi" "Z_aoChan"() -> (w293:tag)
        n96 = property on="generator_enable" class="Bool (strict)"("Value"=FALSE ("Generator  output")) -> ()  [unwired: 2 in, 2 out]
        n97 = global read "GLOBAL_VAR.vi" "COM_MWgenerator"() -> (w290:string)
        n98 = global read "GLOBAL_VAR.vi" "APD_counter_trigger_out"() -> (w292:tag)
        n99 = Build Array(w295, w294, w293) -> (w303:tag[])
        n100 = property on="File name" class="Str"("Value"="" ("File name")) -> ()  [unwired: 2 in, 2 out]
        n101 = call <vilib>:"DAQmx Flatten Channel String.vi"("names in"=w303) -> ("names out"=w302:string)  [unwired: 13 in, 1 out]
        n102 = call "Init_Hittite.vi"("Serial configuration"=T5 {"Baud Rate"=9600, "Parity"=0, "Data Bits"=8, "Stop Bits"=10, "Flow Control"=0} ("Serial Configuration"), "Com_port"=w290, "Trigger_channel"=w292) -> ("Hittite_com"=w299:refnum<visa-resource-name>, "Trigger_out"=w298:refnum<k21>, "error out"=w300:errorcluster)  [unwired: 3 in]
        n103 = call-poly <vilib>:"DAQmx Create Virtual Channel.vi"("maximum value"=10.0, "minimum value"=-10.0, "physical channels"=w302) -> ("task out"=w304:refnum<k21>)  [unwired: 11 in, 1 out]
        n104 = call-poly <vilib>:"DAQmx Create Virtual Channel.vi"("high ticks"=u32 2, "low ticks"=u32 2, "counter"=tag "Dev1/ctr1", "source of ticks"=tag "/Dev1/100MHzTimebase", "idle state"=w317, "initial delay"=u32 2) -> ("task out"=w308:refnum<k21>)  [unwired: 8 in, 1 out]
        n105 = global read "GLOBAL_VAR.vi" "APD_signal"() -> (w291:tag)
        n106 = call <vilib>:"DAQmx Start Task.vi"("task/channels in"=w304) -> ("task out"=w301:refnum<k21>)  [unwired: 13 in, 1 out]
        n107 = call-poly <vilib>:"DAQmx Trigger.vi"("task/channels in"=w308, "source"=w291, "edge"=w313) -> ("task out"=w312:refnum<k21>)  [unwired: 11 in, 1 out]
        n108 = property class="DAQmx Trigger"(reference=w312, "Start.Retriggerable"=TRUE) -> (reference out=w310:refnum<k21>)  [unwired: 1 in, 1 out]
        n109 = call <vilib>:"DAQmx Start Task.vi"("task/channels in"=w310) -> ("task out"=w307:refnum<k21>)  [unwired: 13 in, 1 out]
      }
      frame "stand-by", Default {
        n110 = event shown="[1] \"generator_enable\": Value Change" {
          selector: _ -> [_ _ _ _]
          dyn-events: _ -> [_ _ _ _]
          timeout: 10 -> [_ _ _ _]
          tunnel: w345 -> [w365 _ w446 _]
          tunnel: w343 -> [w361 _ w449 _]
          tunnel: w341 -> [w356 w369 w451 w458]
          tunnel: [w356 _ w451 w458] -> w340
          tunnel: [w355 w370 w450 w459] -> w338
          tunnel: w339 -> [w355 w371 w450 w459]
          tunnel: [_ w369 _ _] -> _
          tunnel: w327 -> [_ _ w434 _]
          tunnel: w337 -> [_ _ w431 _]
          tunnel: w336 -> [_ _ w428 _]
          tunnel: w335 -> [_ _ w423 _]
          tunnel: w334 -> [_ _ w418 _]
          tunnel: w333 -> [_ _ w401 _]
          tunnel: w332 -> [_ _ w400 _]
          tunnel: w331 -> [_ _ w399 _]
          tunnel: w330 -> [_ _ w398 _]
          tunnel: w329 -> [w354 w367 w380 w457]
          tunnel: [w354 w366 w380 w457] -> w328
          event "Intensity Graph": Cursor Move {
            n111 = event-data() -> ()  [unwired: 1 in, 1 out]
            n112 = property on="Intensity Graph" class="IntGraph (strict)"() -> ("Cursor.Cursor Y"=w363:dbl, "Cursor.Cursor X"=w359:dbl)  [unwired: 2 in, 2 out]
            n113 = Round Toward -Infinity(1:w363) -> (0:w360:dbl)
            n114 = Decrement(x=w360) -> (x-1=w362:dbl)
            n115 = local write "Run"(w360) -> ()
            n116 = Index Array(array=w361, index (row)=w362) -> (element=w364:ext[])  [unwired: 1 in]
            n117 = Bundle(w365, w364) -> (w357:cluster{ext[], ext[]})  [unwired: 1 in]
            n118 = property on="Histogram" class="XYGraph (strict)"("Cursor.Cursor X"=w359) -> ()  [unwired: 2 in, 2 out]
            n119 = Build Array(w357, w356) -> (w358:cluster{ext[], ext[]}[])
            n120 = local write "Histogram"(w358) -> ()
          }
          event "generator_enable": Value Change {
            n121 = event-data() -> ("NewVal"=w368:bool)  [unwired: 1 in]
            n122 = case shown="False" w368 {
              tunnel: w371 -> [w375 w379]
              tunnel: [w374 w378] -> w370
              tunnel: w367 -> [w373 w377]
              tunnel: [w372 w376] -> w366
              frame False {
                n123 = call-poly <instrlib>:"Source Output.vi"("error in"=w373, "T2100 Address IN"=w375) -> ("error out"=w372:errorcluster, "T2100 Address OUT"=w374:refnum<visa-resource-name>)  [unwired: 8 in]
              }
              frame True {
                n124 = call-poly <instrlib>:"Source Output.vi"("error in"=w377, "T2100 Address IN"=w379) -> ("error out"=w376:errorcluster, "T2100 Address OUT"=w378:refnum<visa-resource-name>)  [unwired: 8 in]
              }
            }
          }
          event "Save": Value Change {
            n125 = event-data() -> ()  [unwired: 1 in, 6 out]
            n126 = Number To Fractional String(number=w434, precision (6)=i16 0) -> (F-format string=w435:string)  [unwired: 2 in]
            n127 = Number To Fractional String(number=w431, precision (6)=i16 0) -> (F-format string=w432:string)  [unwired: 2 in]
            n128 = Number To Fractional String(number=w428, precision (6)=i16 0) -> (F-format string=w429:string)  [unwired: 2 in]
            n129 = Number To Fractional String(number=w423, precision (6)=i16 3) -> (F-format string=w425:string)  [unwired: 2 in]
            n130 = Concatenate Strings("Step size [Hz] = ", w435, "\r\n") -> (w397:string)
            n131 = Concatenate Strings("Freq start [Hz] = ", w429, "\r\n") -> (w395:string)
            n132 = Concatenate Strings("Dwell time [s] = ", w425, "\r\n") -> (w394:string)
            n133 = Concatenate Strings("Freq stop [Hz] = ", w432, "\r\n") -> (w396:string)
            n134 = Concatenate Strings(w397, w396, w395, w394) -> (w390:string)
            n135 = Get Date/Time In Seconds() -> (seconds since 1Jan1904=w456:timestamp)
            n136 = Format Date/Time String(time format string (%c)="%Y-%m-%d_%H-%M-%S", seconds (now)=w456) -> (date/time string=w455:string)  [unwired: 1 in]
            n137 = Number To Fractional String(number=w418, precision (6)=i16 0) -> (F-format string=w420:string)  [unwired: 2 in]
            n138 = Number To Fractional String(number=w401, precision (6)=i16 3) -> (F-format string=w412:string)  [unwired: 2 in]
            n139 = Number To Fractional String(number=w400, precision (6)=i16 3) -> (F-format string=w409:string)  [unwired: 2 in]
            n140 = Number To Fractional String(number=w399, precision (6)=i16 3) -> (F-format string=w403:string)  [unwired: 2 in]
            n141 = Concatenate Strings(w455, ".dsp") -> (w383:string)
            "File name" <- w383
            n142 = Concatenate Strings("Power [dBm] = ", w420, "\r\n") -> (w389:string)
            n143 = Concatenate Strings("Position X [V] = ", w412, "\r\n") -> (w388:string)
            n144 = Concatenate Strings("Position Y [V] = ", w409, "\r\n") -> (w387:string)
            n145 = Concatenate Strings("Position Z [V] = ", w403, "\r\n") -> (w386:string)
            n146 = Concatenate Strings("D:\\Data\\raw data\\", w383) -> (w381:string)
            n147 = Array To Spreadsheet String(array=w446, 3:"%.0f" ("format string")) -> (spreadsheet string=w445:string)  [unwired: 1 in]
            n148 = Array To Spreadsheet String(array=w449, 3:"%.3f" ("format string")) -> (spreadsheet string=w443:string)  [unwired: 1 in]
            n149 = String To Path(string=w381) -> (path=w452:path)
            n150 = Number To Fractional String(number=w398, precision (6)=i16 0) -> (F-format string=w417:string)  [unwired: 2 in]
            n151 = Concatenate Strings(w445, "\r\n", w443) -> (w392:string)
            n152 = Concatenate Strings("Repetitions = ", w417, "\r\n") -> (w385:string)
            n153 = Concatenate Strings(w390, w389, w388, w387, w386, w385, "\r\n") -> (w391:string)
            n154 = Concatenate Strings(w391, w392) -> (w393:string)
            n155 = call <vilib>:"Write Characters To File.vi"("character string"=w393, "file path (dialog if empty)"=w452) -> ()  [unwired: 3 in, 1 out]
          }
          event Timeout {
            n156 = event-data() -> ()  [unwired: 1 in, 3 out]
          }
        }
        n157 = Not(x="start") -> (.not. x?=w351:bool)
        n158 = Select(t=w353, s=w351, f=T4."Set Variables") -> (s? t:f=w352:T3)
      }
    }
    n159 = Not(x="stop") -> (.not. x?=w47:bool)
    n160 = Select(t=w45, s=w47, f=T4."close") -> (s? t:f=w23:T3)
    n161 = case shown="Error" w22 {
      tunnel: [w61 T3."Error Check"] -> w24
      tunnel: w23 -> [w61 _]
      frame No Error {
      }
      frame Error {
      }
    }
  }
